vi "TF conditions and checking.vi"(0 "Input Points":dbl[](array[numeric]) format="%.2f", 1 "Transfer Functions":T1(array[cluster]) {"Denominator" format="%.2f"; "Numerator" format="%.2f"}) -> (2 "internal states":cluster{dbl[]}[](array[cluster]) {"?" format="%.2f"}, 3 "additive constants":dbl[](array[numeric]) format="%.2f", 4 "previous samples":dbl[](array[numeric]) format="%.2f", 5 "numerators":cluster{"Numerator new":dbl[]}[](array[cluster]) {"Numerator new" format="%.2f"}, 6 "denominators":cluster{dbl[]}[](array[cluster]) {"?" format="%.2f"}, 7 "gains":dbl[](array[numeric]) format="%.2f")   [LabVIEW 2017, in "NI_AdvCtrl_continuous linear.lvlib"]
doc: "LabVIEW no longer supports this VI. You can obtain similar functionality by installing the LabVIEW Simulation Module."
uses:
  <vilib>/addons/control/advanced/NI_AdvCtrl_continuous linear.lvlib
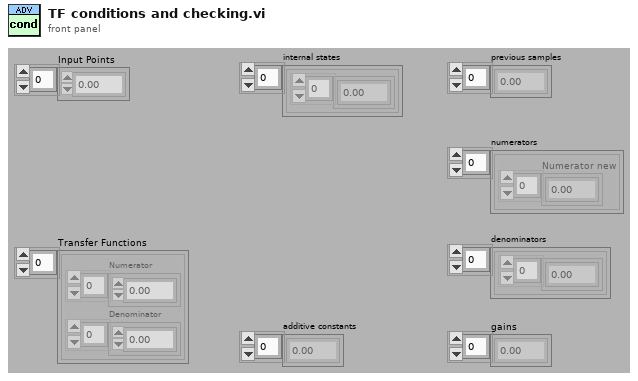
[diagram p1: front panel]
types:
  T1 = cluster{"Numerator":dbl[], "Denominator":dbl[]}[]
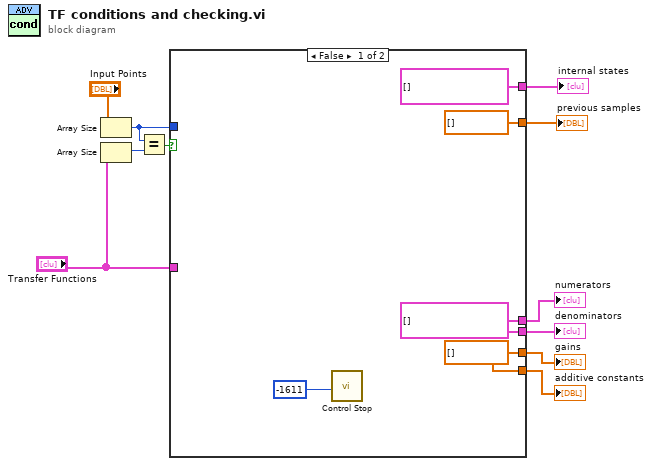
[diagram p0: block diagram]
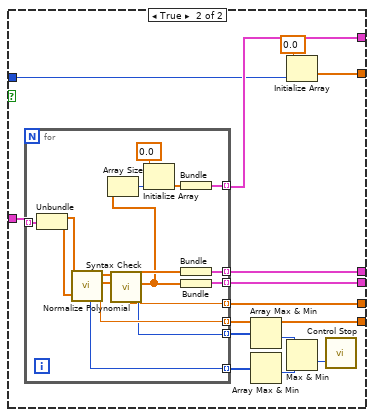
[diagram p2: hidden frame]
diagram:
  n1 = Array Size(array="Input Points") -> (size(s)=w9:i32)
  n2 = Array Size(array="Transfer Functions") -> (size(s)=w10:i32)
  n3 = Equal?(x=w9, y=w10) -> (x = y?=w11:bool)
  n4 = case shown="False" w11 {
    tunnel: [w13 w30] -> w1
    tunnel: [w13 w29] -> w2
    tunnel: [w14 w28] -> w3
    tunnel: [w14 w27] -> w4
    tunnel: [cluster{dbl[]}[] [] w26] -> w5
    tunnel: [dbl[] [] w19] -> w7
    tunnel: "Transfer Functions" -> [_ w18]
    tunnel: w9 -> [_ w17]
    frame False {
      w13 = dbl[] []
      w14 = cluster{"Numerator new":dbl[]}[] []
      n5 = call <vilib>:"Control Stop.vi"("error"=-1611 ("f")) -> ()  [unwired: 2 out]
    }
    frame True {
      n6 = for {
        tunnel: [w47] -> w24 mode=indexing
        tunnel: [w46] -> w30 mode=indexing
        tunnel: [w43] -> w25 mode=indexing
        tunnel: [w42] -> w29 mode=indexing
        tunnel: [w34] -> w28 mode=indexing
        tunnel: [w33] -> w27 mode=indexing
        tunnel: [w37] -> w26 mode=indexing
        tunnel: w18 -> [w36] mode=indexing
        n7 = Unbundle(w36) -> ("Numerator"=w35:dbl[], "Denominator"=w32:dbl[])
        n8 = call <vilib>:"Normalize Polynomial.vi"("Numerator"=w35, "Denominator"=w32) -> ("Numerator new"=w44:dbl[], "Denominator new"=w45:dbl[], "additive constant"=w46:dbl, "error"=w47:i32)
        n9 = call <vilib>:"Syntax Check.vi"("Denominator"=w45, "Numerator"=w44) -> ("error"=w43:i32, "gain"=w42:dbl, "Denominator new"=w31:dbl[], "Numerator new"=w41:dbl[])  [unwired: 1 out]
        n10 = Array Size(array=w31) -> (size(s)=w39:i32)
        n11 = Initialize Array(0.0, w39) -> (w38:dbl[])
        n12 = Bundle(w38) -> (w37:cluster{dbl[]})  [unwired: 1 in]
        n13 = Bundle("Numerator new"=w41) -> (w34:cluster{"Numerator new":dbl[]})  [unwired: 1 in]
        n14 = Bundle("Denominator new"=w31) -> (w33:cluster{"Denominator new":dbl[]})  [unwired: 1 in]
      }
      n15 = Array Max & Min(array=w25) -> (min value=w23:i32)  [unwired: 3 out]
      n16 = Array Max & Min(array=w24) -> (min value=w22:i32)  [unwired: 3 out]
      n17 = Initialize Array(0.0 ("Element Data"), w17) -> (w19:dbl[])
      n18 = Max & Min(x=w23, y=w22) -> (min(x,y)=w21:i32)  [unwired: 1 out]
      n19 = call <vilib>:"Control Stop.vi"("error"=w21) -> ()  [unwired: 2 out]
    }
  }
  "previous samples" <- w7
  "internal states" <- w5
  "denominators" <- w4
  "numerators" <- w3
  "gains" <- w2
  "additive constants" <- w1
